vi "VoorbeeldVanProject_vi.vi"() -> ()   [LabVIEW 2019]
panel:
  out "Boolean 2":bool
  in  "Boolean":bool
  in  "stop":bool
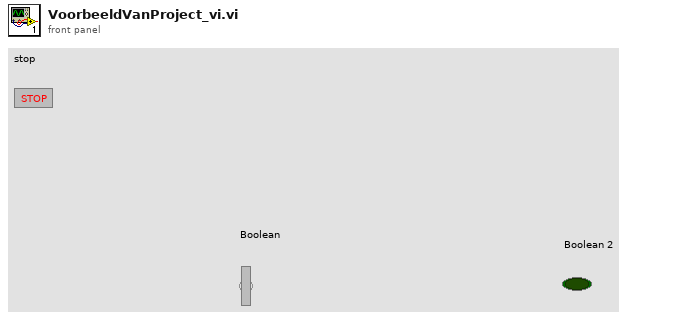
[diagram p1: front panel]
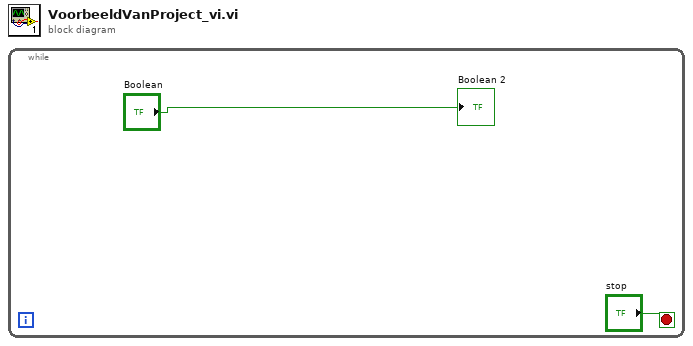
[diagram p0: block diagram]
diagram:
  n1 = while {
    stop <- "stop" stop-if-true
    "Boolean 2" <- "Boolean"
  }
